vi "Panel.vi"(8 "error in (no error)":errorcluster, 11 "Target Step in":refnum<class "Target Step.lvclass">) -> ()   [LabVIEW 2018, in "Temp Recipe.lvlib" / "Target Step.lvclass"]
uses:
  Target Step.lvclass
  C:/dev/source/Systems/NI Week/Temperature Recipe/Temp Recipe/Recipe Step/Recipe Step.lvclass
  C:/dev/source/Libraries/OOPanel/OOPanel/Panel/Panel.lvclass
  Libraries/OOPanel/OOPanel/Panel/Panel.lvclass
  Recipe Step/Recipe Step.lvclass
  Libraries/OOPanel/OOPanel/PanelArray/PanelArray.lvclass
panel:
  in  "Duration":dbl format="%#.6f Hours"
  in  "Setpoint":dbl format="%.1f °F"
  in  "Remove Button":bool
  in  "Down Button":bool
  in  "Up Button":bool
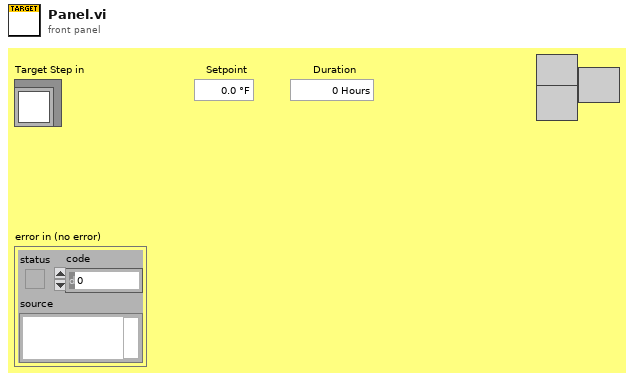
[diagram p1: front panel]
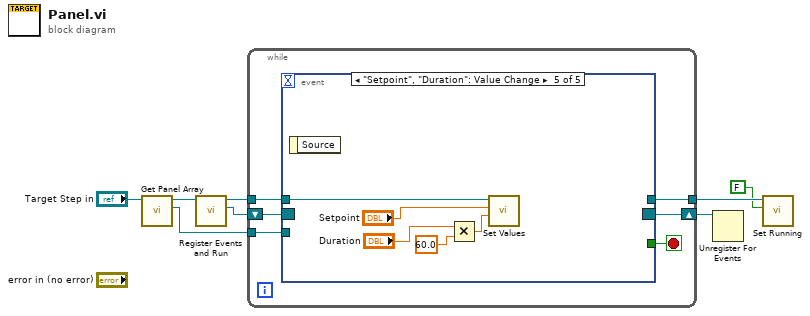
[diagram p0: block diagram]
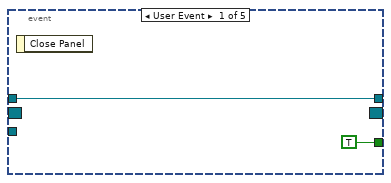
[diagram p2: hidden frame]
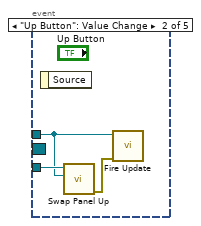
[diagram p3: hidden frame]
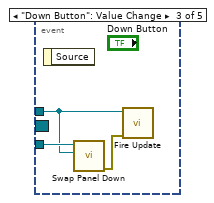
[diagram p4: hidden frame]
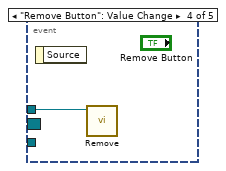
[diagram p5: hidden frame]
diagram:
  n1 = call "Get Panel Array.vi"("Recipe Step in"="Target Step in") -> ("PanelArray"=w1:refnum<class "PanelArray.lvclass">, "Recipe Step out"=w2:refnum<class "Target Step.lvclass">)  [unwired: 8 in, 1 out]
  n2 = call "Register Events and Run.vi"("Panel in"=w2) -> ("Event Registration Refnum"=w7:refnum<event-registration>, "Panel out"=w8:refnum<class "Target Step.lvclass">)  [unwired: 8 in, 1 out]
  n3 = while {
    tunnel: w8 -> [w13]
    shift-right: [w11] -> w6
    shift-left: w7 -> [w14]
    tunnel: [w10] -> w5
    tunnel: w1 -> [w9]
    stop <- w12 stop-if-true
    n4 = event shown="[4] \"Setpoint\", \"Duration\": Value Change" {
      selector: w14 -> [_ _ _ _ _]
      dyn-events: [_ _ _ _ _] -> w11
      timeout: _ -> [_ _ _ _ _]
      tunnel: w13 -> [w15 w18 w21 w23 w28]
      tunnel: [TRUE _ _ _ _] -> w12
      tunnel: [w15 _ _ _ _] -> w10
      tunnel: w9 -> [_ w19 w22 _ _]
      event User Event {
        n5 = event-data() -> ()  [unwired: 1 in, 1 out]
      }
      event "Up Button": Value Change {
        n6 = event-data() -> ()  [unwired: 1 in, 1 out]
        n7 = call "Swap Panel Up.vi"("Panel"=w18, "PanelArray in"=w19) -> ("error out"=w17:errorcluster)  [unwired: 8 in, 1 out]
        n8 = call "Fire Update.vi"("error in (no error)"=w17, "Recipe Step in"=w18) -> ()  [unwired: 8 in, 2 out]
      }
      event "Down Button": Value Change {
        n9 = event-data() -> ()  [unwired: 1 in, 1 out]
        n10 = call "Swap Panel Down.vi"("Panel"=w21, "PanelArray in"=w22) -> ("error out"=w20:errorcluster)  [unwired: 8 in, 1 out]
        n11 = call "Fire Update.vi"("error in (no error)"=w20, "Recipe Step in"=w21) -> ()  [unwired: 8 in, 2 out]
      }
      event "Remove Button": Value Change {
        n12 = event-data() -> ()  [unwired: 1 in, 1 out]
        n13 = call "Remove.vi"("Recipe Step in"=w23) -> ()  [unwired: 9 in, 2 out]
      }
      event "Setpoint", "Duration": Value Change {
        n14 = event-data() -> ()  [unwired: 1 in, 1 out]
        n15 = Multiply(x="Duration", y=60.0) -> (x*y=w26:dbl)
        n16 = call "Set Values.vi"("Settle Time"=w26, "Step Temp"="Setpoint", "Target Step in"=w28) -> ()  [unwired: 7 in, 2 out]
      }
    }
  }
  n17 = Unregister For Events(event registration refnum=w6) -> ()  [unwired: 1 in, 1 out]
  n18 = call "Set Running.vi"("Running"=FALSE, "Panel in"=w5) -> ()  [unwired: 8 in, 2 out]
